vi "StepperMotor.vi"(8 "error in":errorcluster, 9 "Direction":bool, 10 "Time between steps (ms)":i32=1, 11 "Steps":i64=1) -> (0 "error out":errorcluster)   [LabVIEW 2021]
doc: "André Romero - 2020\nandretec@ifsc.usp.br"
panel:
  # "DRV8825 Stepper Motor"
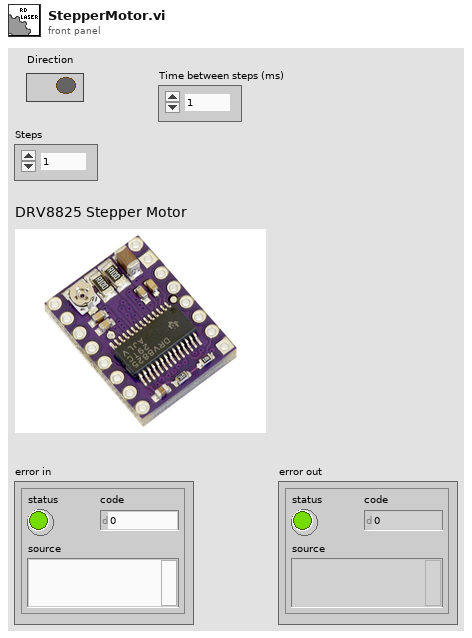
[diagram p1: front panel]
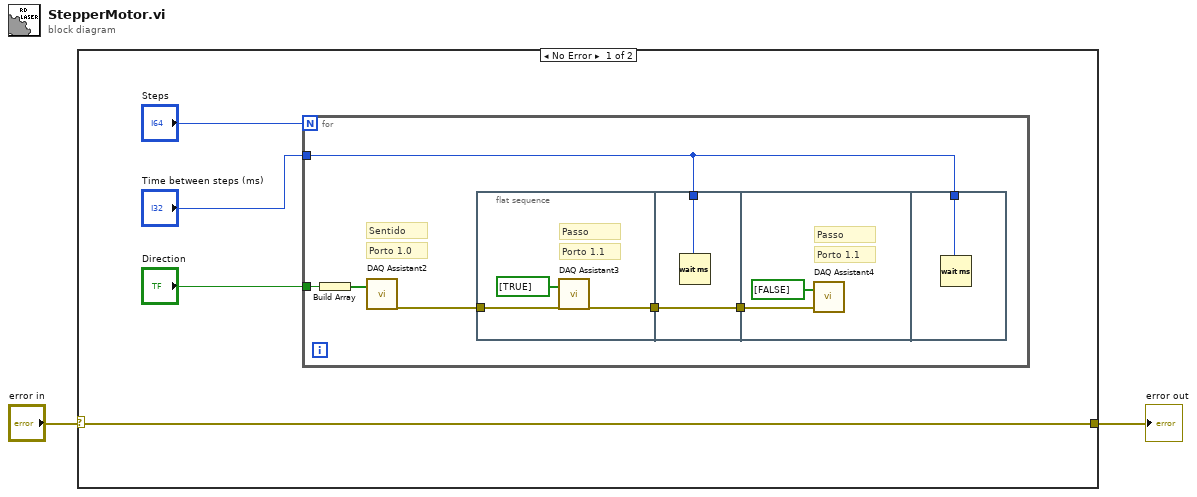
[diagram p0: block diagram]
diagram:
  n1 = case shown="No Error" "error in" {
    selector: "error in" -> [w3 w21]
    tunnel: [w3 w21] -> w1
    frame No Error {
      n2 = for {
        N: "Steps" -> [_]
        tunnel: "Direction" -> [w11]
        tunnel: "Time between steps (ms)" -> [w9]
        # "Sentido"
        # "Porto 1.0"
        n3 = Build Array(w11) -> (w12:bool[])
        n4 = call "DAQ Assistant2"("data"=w12) -> ("error out"=w10:errorcluster)  [unwired: 17 in, 1 out]
        n5 = flat-sequence {
          tunnel: w10 -> [w15]
          tunnel: [w13] -> w8
          tunnel: w9 -> [w17]
          tunnel: w8 -> [w16]
          tunnel: [w16] -> w7
          tunnel: w7 -> [w18]
          tunnel: w9 -> [w20]
          frame #0 {
            # "Passo"
            # "Porto 1.1"
            n6 = call "DAQ Assistant3"("data"=bool[] [TRUE], "error in"=w15) -> ("error out"=w13:errorcluster)  [unwired: 16 in, 1 out]
          }
          frame #1 {
            n7 = Wait (ms)(milliseconds to wait=w17) -> ()  [unwired: 1 out]
          }
          frame #2 {
            # "Passo"
            # "Porto 1.1"
            n8 = call "DAQ Assistant4"("data"=bool[] [FALSE], "error in"=w18) -> ()  [unwired: 16 in, 2 out]
          }
          frame #3 {
            n9 = Wait (ms)(milliseconds to wait=w20) -> ()  [unwired: 1 out]
          }
        }
      }
    }
    frame Error {
    }
  }
  "error out" <- w1
